vi "Multi Reader - Read Same Rates - State Machine.vi"(7 "Popup? (F)":bool, 8 "error in (no error)":errorcluster, 10 "Signals in":refnum<class "ISignal.lvclass">[](array[class])) -> (0 "error out":errorcluster)   [LabVIEW 2022 SP3, in "MultiReader.lvlib"]
uses:
  <instrlib>/openDAQ/Examples/MultiReader/MultiReader.lvlib
  <instrlib>/openDAQ/Public/TypeDef/DomainMetadata.ctl
  <instrlib>/openDAQ/Public/Classes/ISignal/ISignal.lvclass
  C:/Program Files (x86)/National Instruments/LabVIEW 2022/instr.lib/openDAQ/Public/Classes/IComponent/IComponent.lvclass
  C:/Program Files (x86)/National Instruments/LabVIEW 2022/instr.lib/openDAQ/Public/Classes/IBaseObject/IBaseObject.lvclass
  <instrlib>/openDAQ/Examples/MultiReader/TypeDef/State.ctl
  <instrlib>/openDAQ/Public/Classes/IInstance/IInstance.lvclass
  C:/Program Files (x86)/National Instruments/LabVIEW 2022/instr.lib/openDAQ/Public/Classes/IDevice/IDevice.lvclass
  <instrlib>/openDAQ/Public/Classes/IDevice/IDevice.lvclass
  <instrlib>/openDAQ/Public/Classes/IMultiReader/IMultiReader.lvclass
  C:/Program Files (x86)/National Instruments/LabVIEW 2022/instr.lib/openDAQ/Public/Classes/IReader/IReader.lvclass
  <instrlib>/openDAQ/Public/TypeDef/daqSampleType.ctl
  <instrlib>/openDAQ/Public/Classes/IMultiReaderStatus/IMultiReaderStatus.lvclass
  C:/Program Files (x86)/National Instruments/LabVIEW 2022/instr.lib/openDAQ/Public/Classes/IReaderStatus/IReaderStatus.lvclass
  <instrlib>/openDAQ/Public/Classes/IBaseObject/Polymorphic/queryInterface/queryDataDescriptorInterface.vi
  <instrlib>/openDAQ/Public/Classes/IMultiReaderBuilder/IMultiReaderBuilder.lvclass
  <instrlib>/openDAQ/Public/Classes/daqCoreTypes/IDict/IDict.lvclass
  <instrlib>/openDAQ/Public/Classes/IBaseObject/IBaseObject.lvclass
  <instrlib>/openDAQ/Public/Classes/IDataDescriptor/IDataDescriptor.lvclass
  <instrlib>/openDAQ/Public/Classes/IEventPacket/IEventPacket.lvclass
  <instrlib>/openDAQ/Public/Classes/daqUtils/daqUtils.lvlib
  <instrlib>/openDAQ/openDAQ.lvlib
  <instrlib>/openDAQ/Public/Classes/IComponent/IComponent.lvclass
  <instrlib>/openDAQ/Public/Classes/IReader/IReader.lvclass
  <instrlib>/openDAQ/Public/Classes/IReaderStatus/IReaderStatus.lvclass
panel:
  in  "Btn:StopMeasurement":bool
  in  "Online Buffer":i32=1000
  in  "Btn:StartMeasurement":bool
  out "Str:SampleRate":string
  in  "Btn:Stop":bool
  out "Iteration":i32
  out "DomainMetadata":T1
  out "Global ID's":string[](array[string])
  out "XY Graph":cluster{dbl[], "Read Buffers out":dbl[]}[](graph)
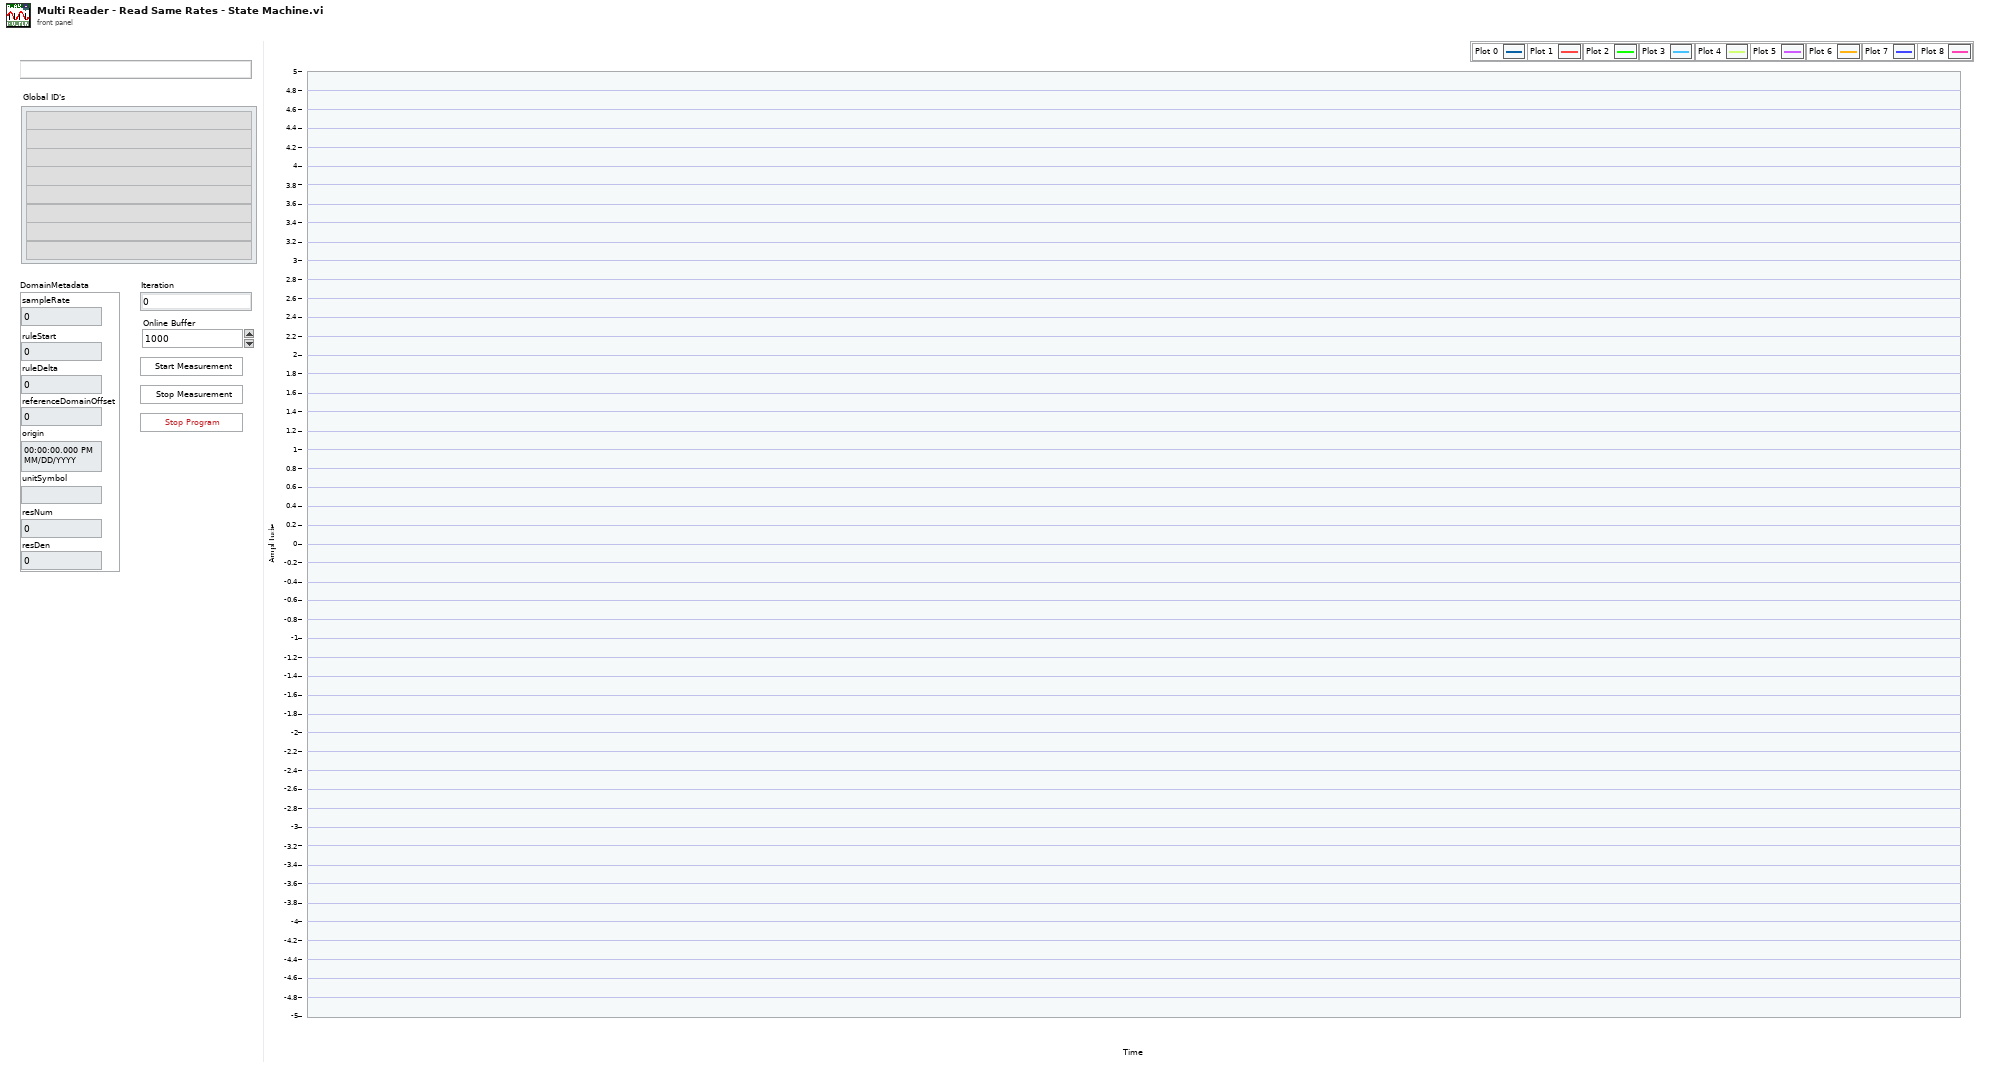
[diagram p1: front panel]
types:
  T1 = typedef "openDAQ.lvlib/DomainMetadata.ctl" = cluster{"sampleRate":i64, "ruleStart":i64, "ruleDelta":i64, "referenceDomainOffset":i64, "origin":timestamp, "unitSymbol":string, "resNum":i64, "resDen":i64}
  T2 = cluster{"Simulator":refnum<class "IInstance.lvclass">, "Instance":refnum<class "IInstance.lvclass">, "ConnectedDevice":refnum<class "IDevice.lvclass">, "Signals":refnum<class "ISignal.lvclass">[], "ChannelCount":i32, "MultiReader":refnum<class "IMultiReader.lvclass">}
  T3 = typedef "MultiReader.lvlib/State.ctl" = enum16{"INIT", "- SIMULATOR.setup", "IDLE", "- DAQ.start", "- DAQ.read", "- DAQ.end", "STOP", "ERROR"}
  T4 = enum16{"init", "read", "set sampleRate", "set ruleStart", "set ruleDelta", "set referenceDomainOffset", "set origin", "set unitSymbol", "set resNum", "set resDen", " calculate sampleRate"}
  T5 = enum8{"Enabled", "Disabled", "Disabled and Grayed Out"}
  T6 = typedef "openDAQ.lvlib/daqSampleType.ctl" = u16
  T7 = typedef "openDAQ.lvlib/ReadStatus.ctl" = u16
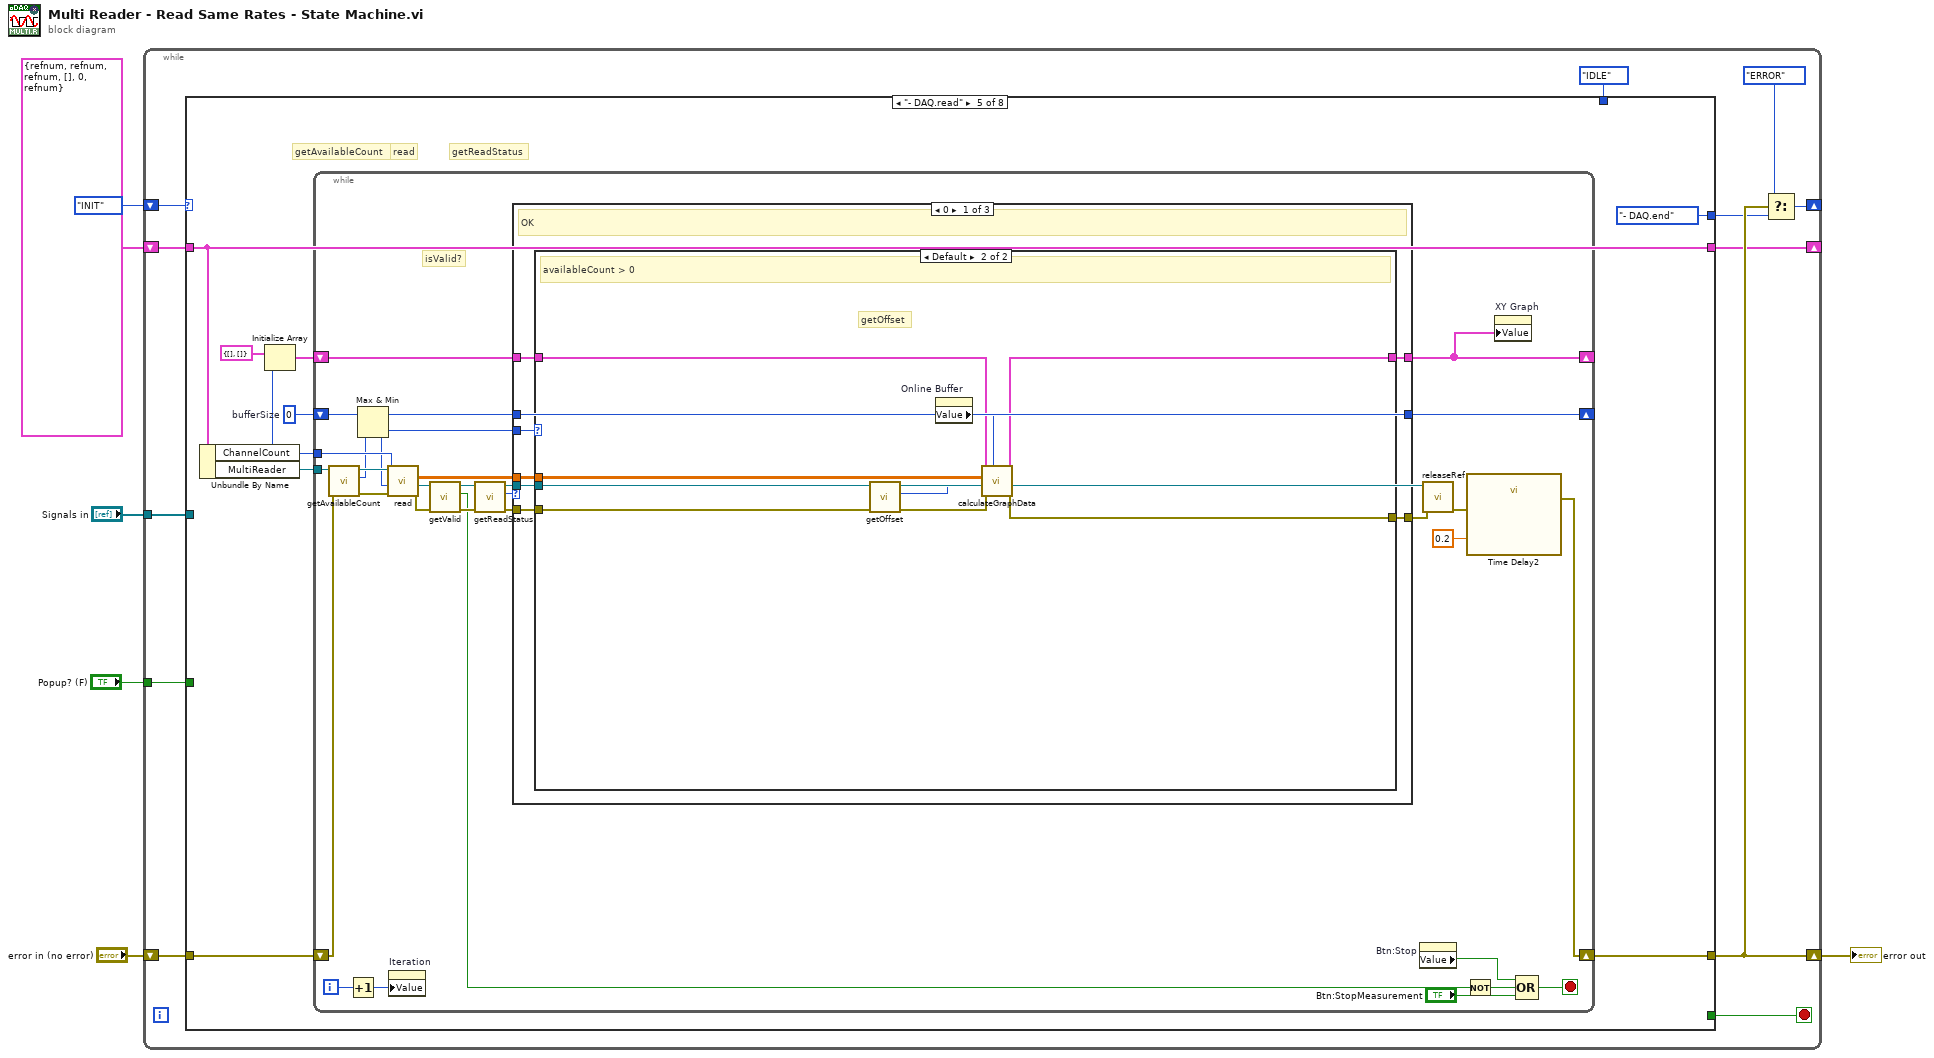
[diagram p0: block diagram]
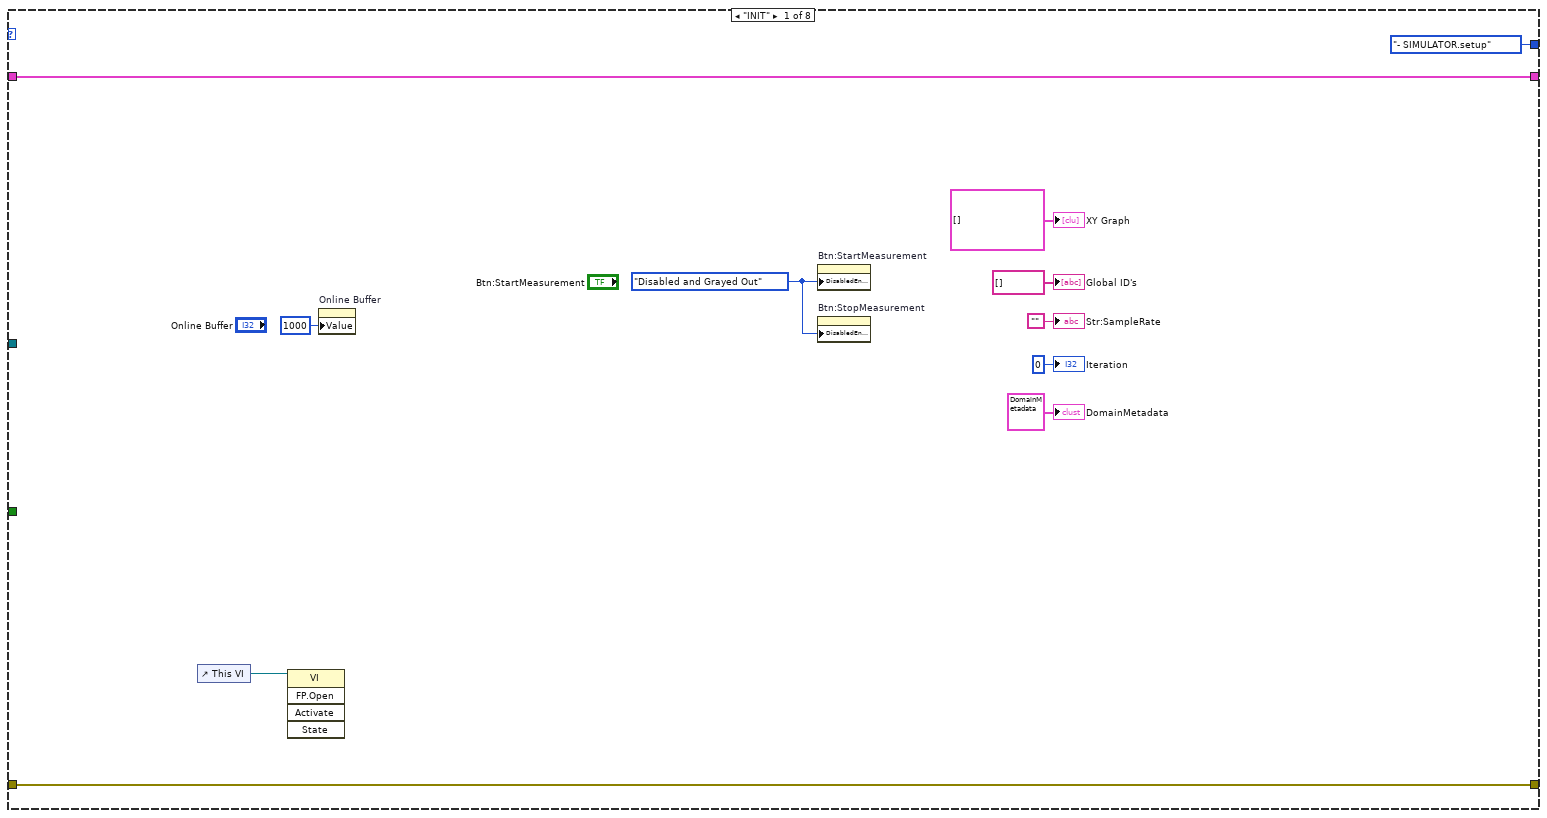
[diagram p2: hidden frame]
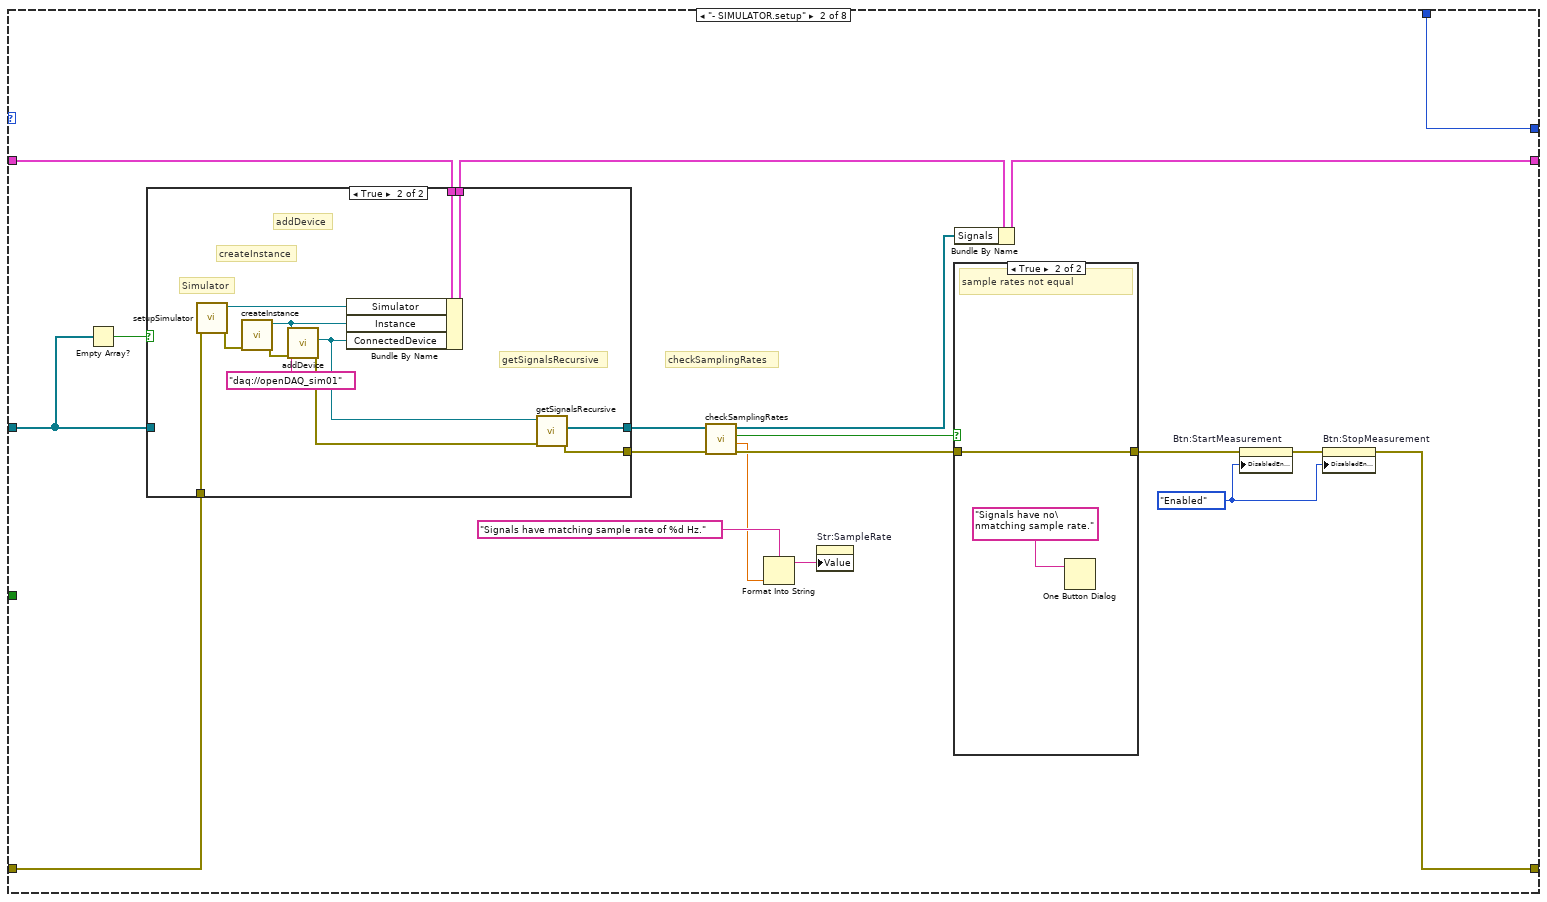
[diagram p3: hidden frame]
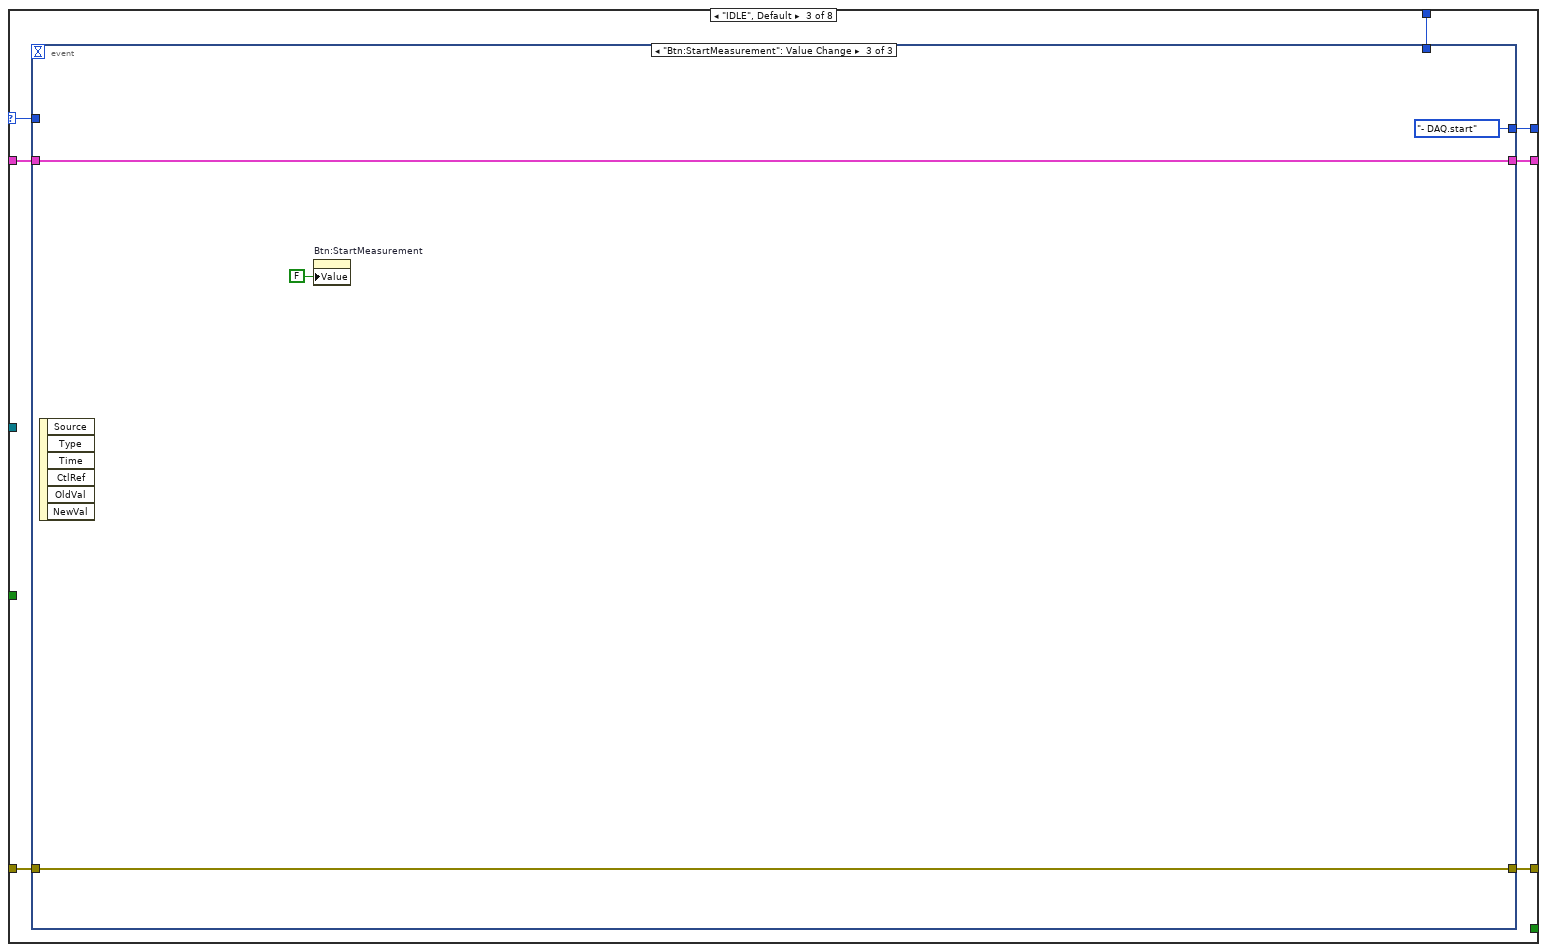
[diagram p6: hidden frame]
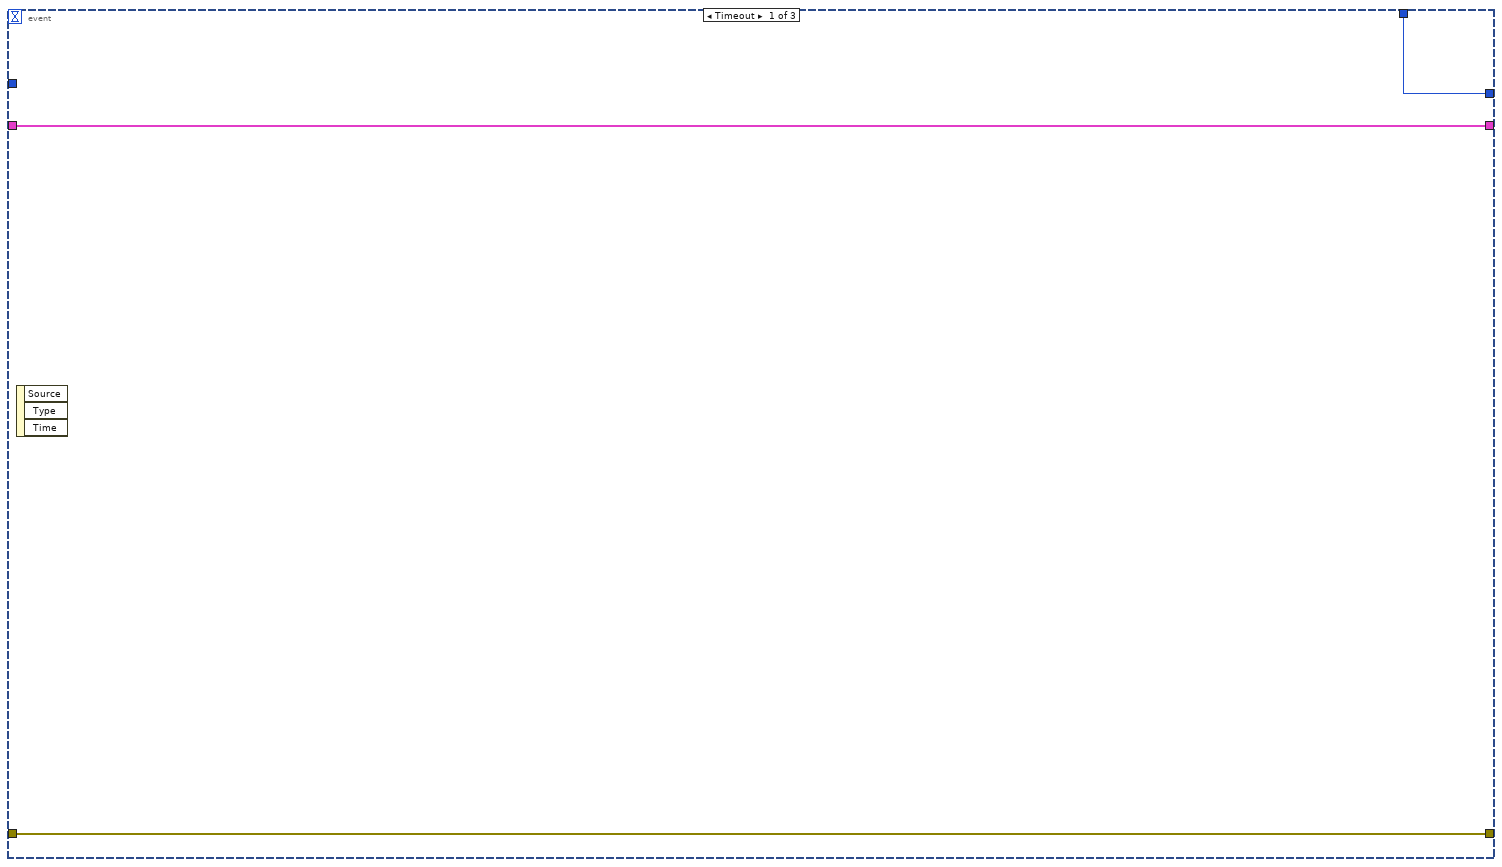
[diagram p7: hidden frame]
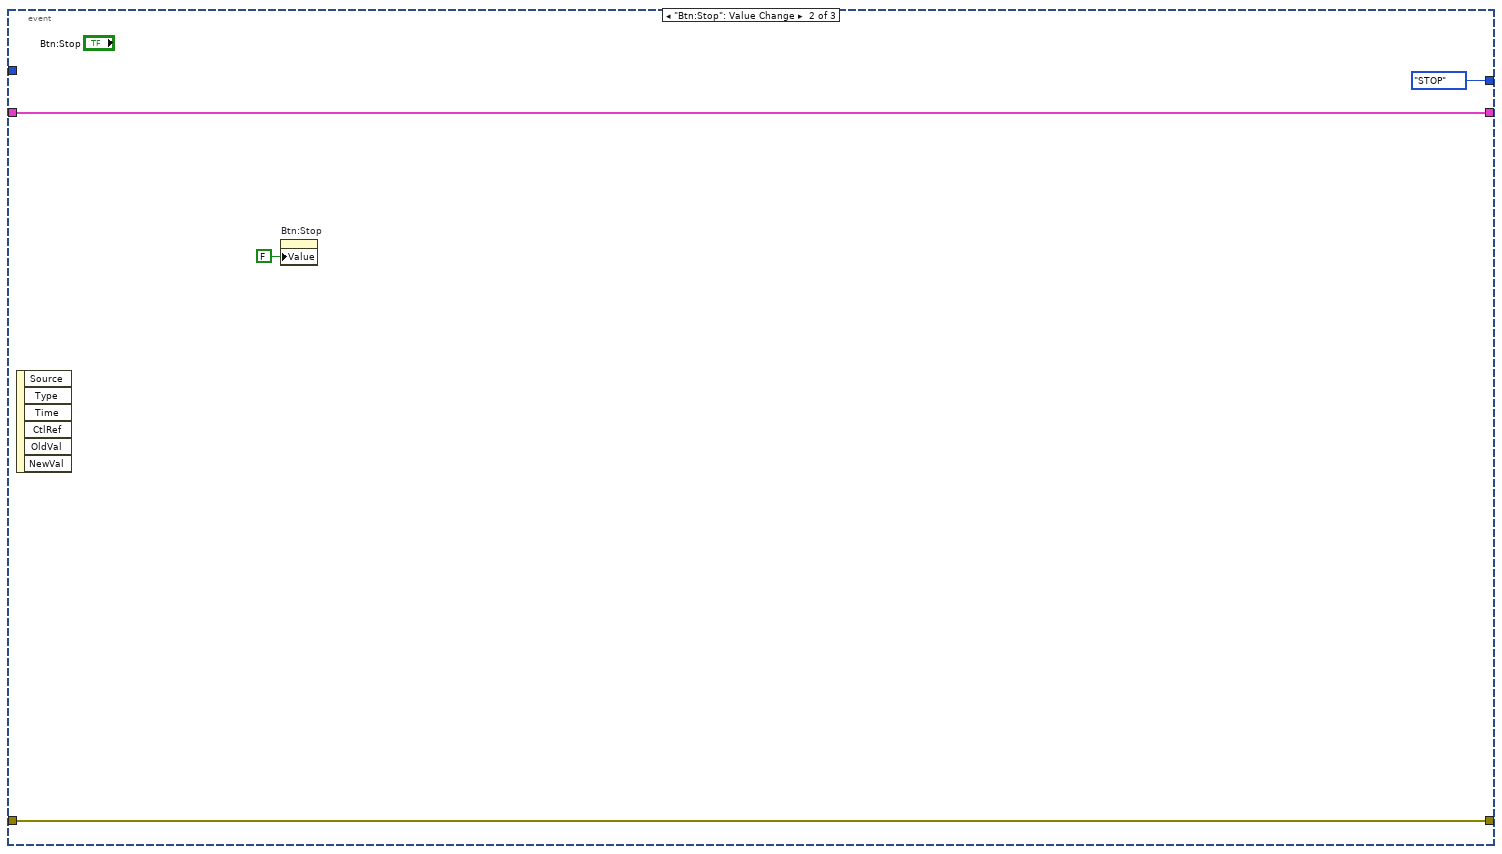
[diagram p8: hidden frame]
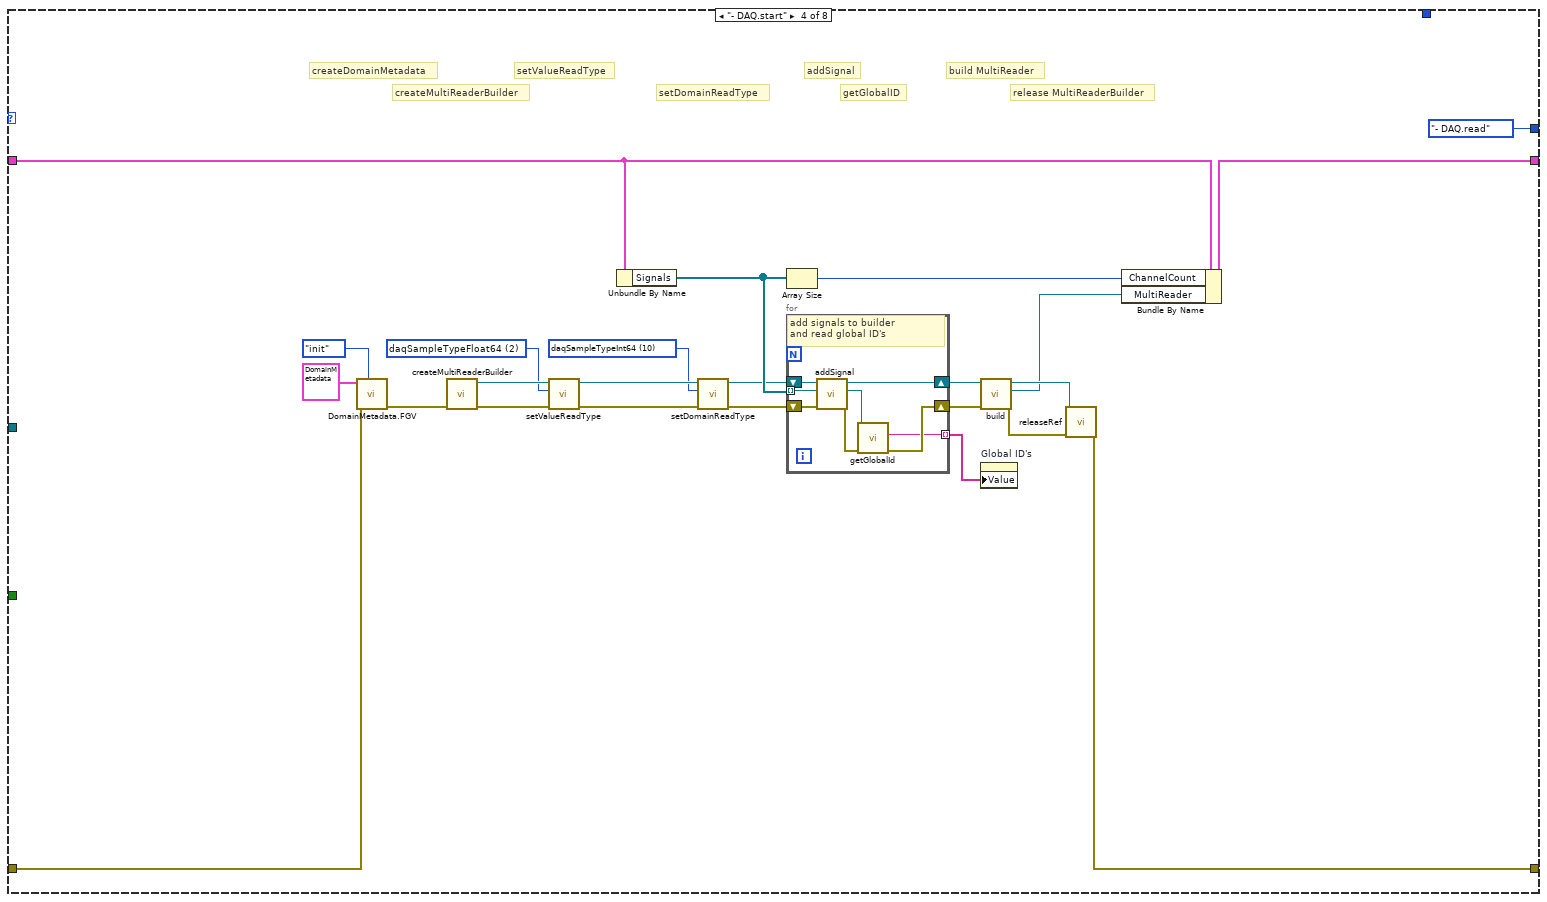
[diagram p9: hidden frame]
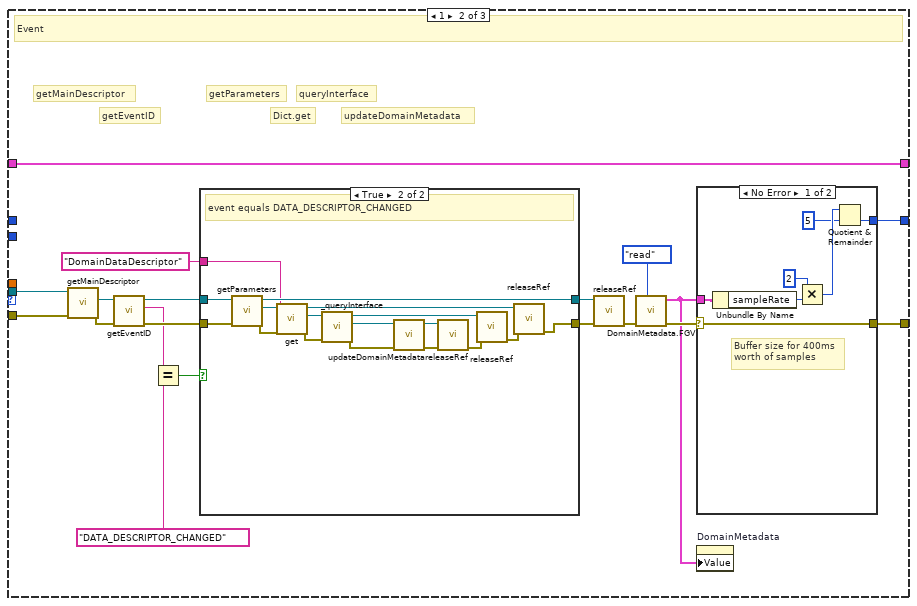
[diagram p11: hidden frame]
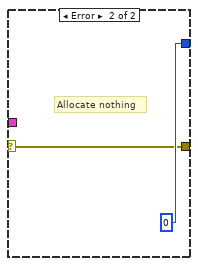
[diagram p12: hidden frame]
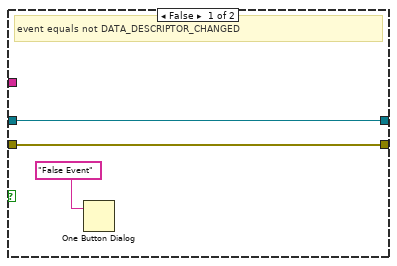
[diagram p13: hidden frame]
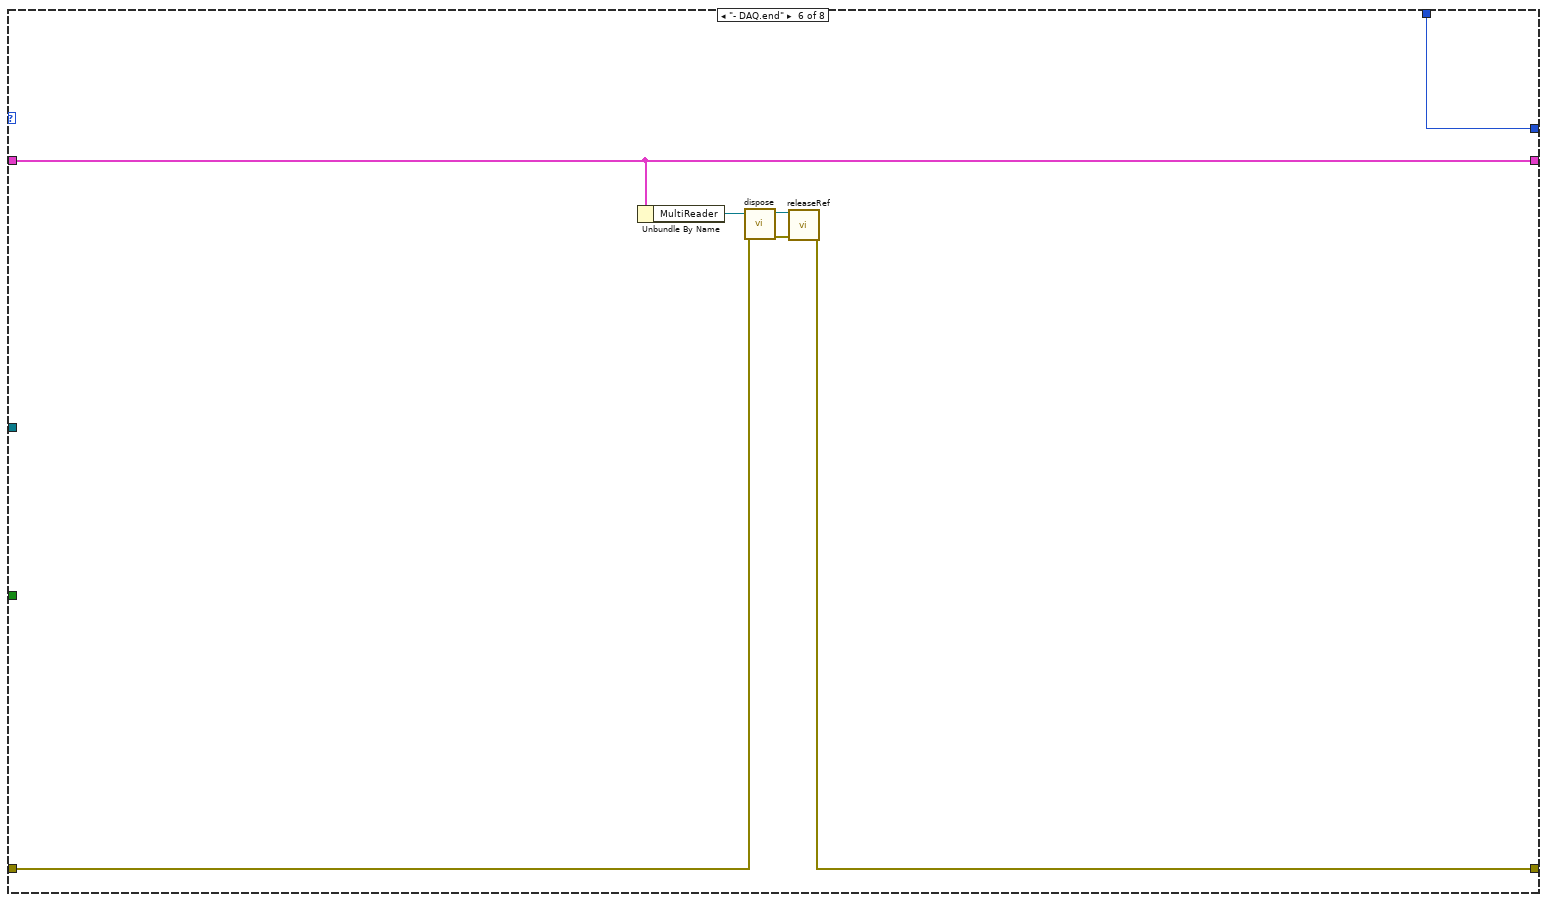
[diagram p15: hidden frame]
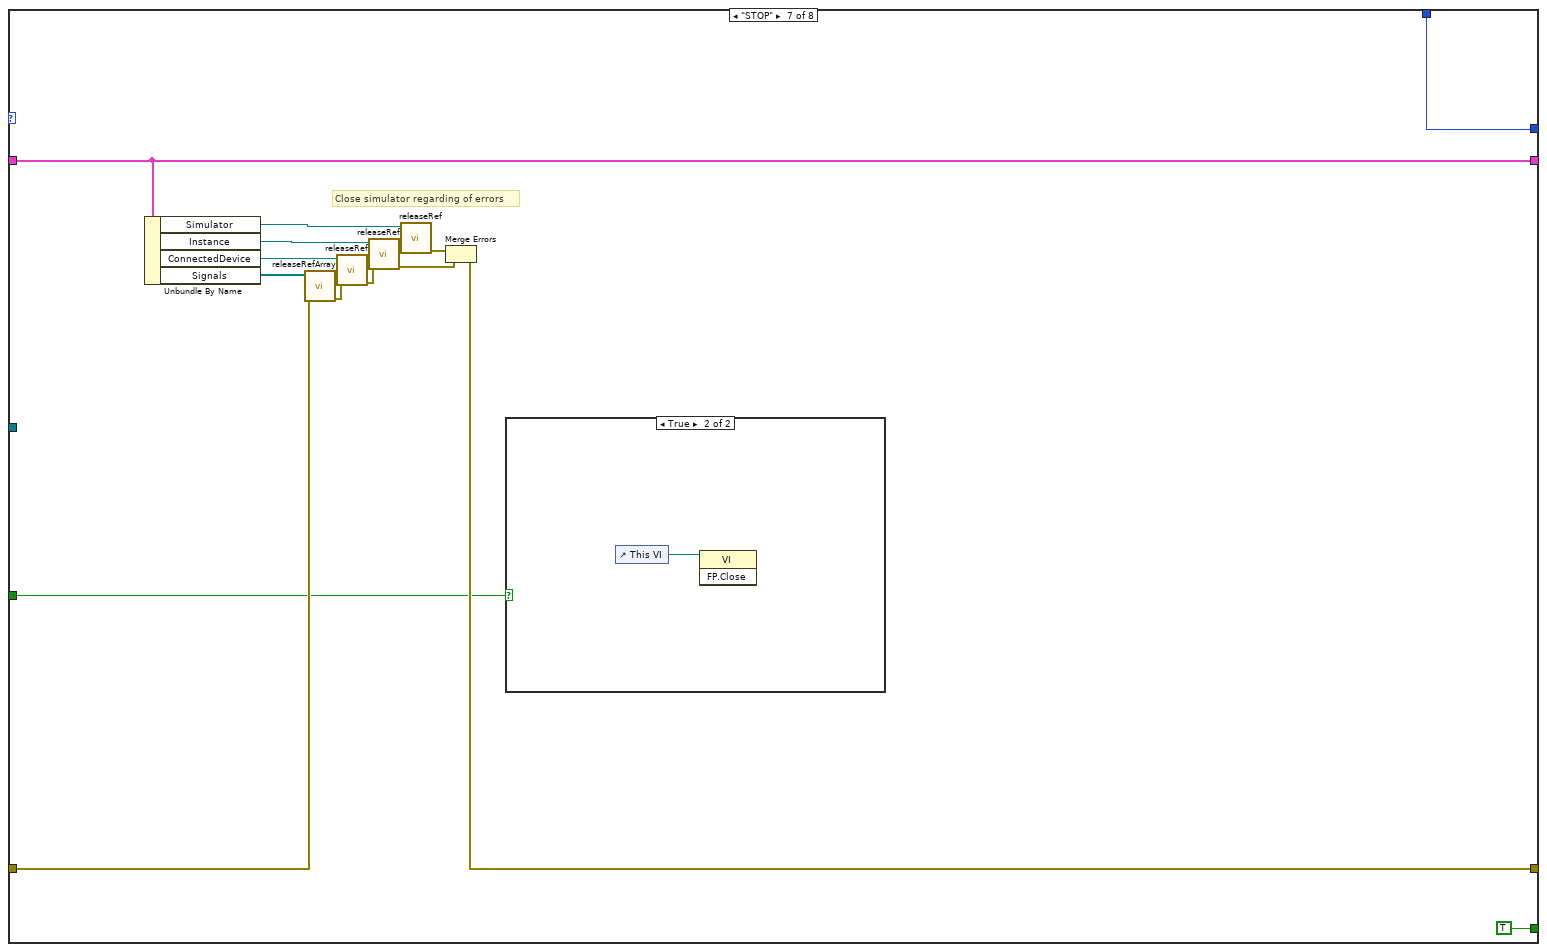
[diagram p16: hidden frame]
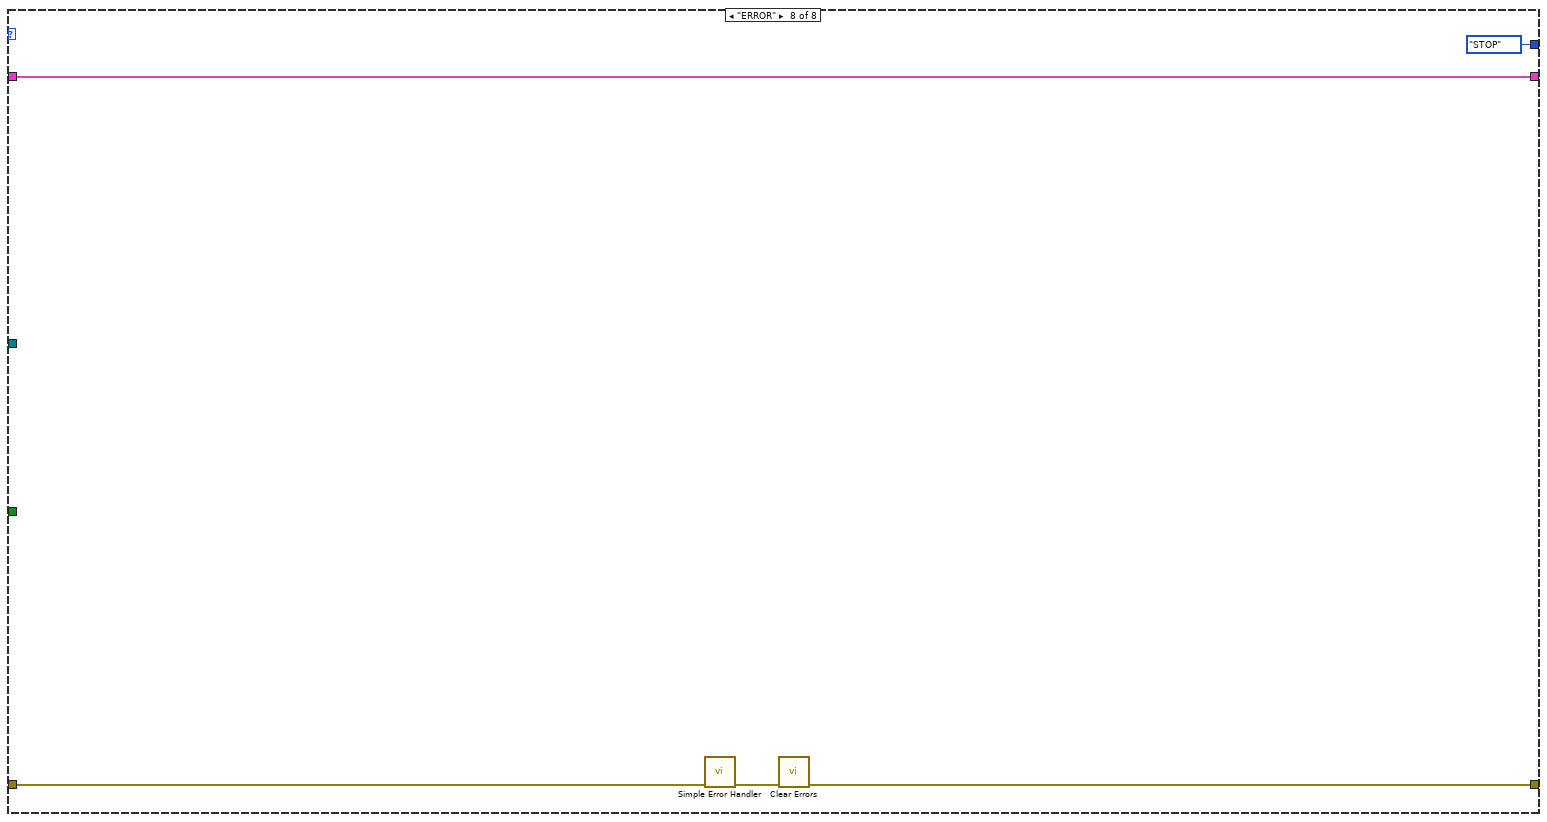
[diagram p18: hidden frame]
diagram:
  n1 = while {
    shift-right: [w11] -> _
    shift-left: State."INIT" -> [w17]
    shift-right: [w18] -> w2
    shift-left: "error in (no error)" -> [w14]
    shift-right: [w12] -> _
    shift-left: T2 {"Simulator"=refnum, "Instance"=refnum, "ConnectedDevice"=refnum, "Signals"=[], "ChannelCount"=0, "MultiReader"=refnum} -> [w13]
    tunnel: "Signals in" -> [w8]
    tunnel: "Popup? (F)" -> [w7]
    stop <- w16 stop-if-true
    n2 = case shown="\"- DAQ.read\"" w17 {
      selector: w17 -> [_ _ w73 _ _ _ _ _]
      tunnel: [State."- SIMULATOR.setup" w47 w71 State."- DAQ.read" State."- DAQ.end" w233 w235 State."STOP"] -> w10
      tunnel: [_ _ _ _ _ _ TRUE _] -> w16
      tunnel: State."IDLE" -> [_ w47 w72 _ _ w233 w235 _]
      tunnel: w14 -> [w22 w48 w70 w93 w123 w229 w237 w251]
      tunnel: [w22 w33 w69 w87 w122 w231 w240 w250] -> w18
      tunnel: w13 -> [w29 w46 w68 w97 w124 w232 w246 w253]
      tunnel: [w29 w41 w67 w85 w124 w232 w246 w253] -> w12
      tunnel: w8 -> [_ w30 _ _ _ _ _ _]
      tunnel: w7 -> [_ _ _ _ _ _ w234 _]
      frame "INIT" {
        w20 = T5."Disabled and Grayed Out" ("Disabled")
        n3 = control-ref of="This VI"() -> (w19:refnum<vi>)
        n4 = invoke class="VI" method="FP.Open"(reference=w19) -> ()  [unwired: 4 in, 5 out]
        n5 = property on="Online Buffer" class="DigNum (strict)"("Value"=1000 ("Online Buffer")) -> ()  [unwired: 2 in, 2 out]
        n6 = property on="Btn:StartMeasurement" class="Bool (strict)"("DisabledEnum"=w20) -> ()  [unwired: 2 in, 2 out]
        n7 = property on="Btn:StopMeasurement" class="Bool"("DisabledEnum"=w20) -> ()  [unwired: 2 in, 2 out]
        "Global ID's" <- string[] [] ("Global ID's")
        "Str:SampleRate" <- "" ("Str:SampleRate")
        "Iteration" <- 0 ("Iteration")
        "XY Graph" <- cluster{dbl[], "Read Buffers out":dbl[]}[] [] ("XY Graph")
        "DomainMetadata" <- T1 {"sampleRate"=0, "ruleStart"=0, "ruleDelta"=0, "referenceDomainOffset"=0, "origin"=timestamp(0 s since 1904-01-01), "unitSymbol"="", "resNum"=0, "resDen"=0} ("DomainMetadata")
      }
      frame "- SIMULATOR.setup" {
        w32 = T5."Enabled" ("Disabled")
        # "checkSamplingRates"
        n8 = Empty Array?(array=w30) -> (empty?=w31:bool)
        n9 = case shown="True" w31 {
          tunnel: w48 -> [w50 w63]
          tunnel: w46 -> [w51 w57]
          tunnel: [w49 w56] -> w45
          tunnel: [w51 w53] -> w42
          tunnel: [w50 w52] -> w36
          tunnel: w30 -> [w49 _]
          frame False {
          }
          frame True {
            # "Simulator"
            # "addDevice"
            # "createInstance"
            # "getSignalsRecursive"
            n10 = call <instrlib>:"setupSimulator.vi"("error in (no error)"=w63) -> ("error out"=w60:errorcluster, "IInstance out"=w59:refnum<class "IInstance.lvclass">)  [unwired: 9 in]
            n11 = call <instrlib>:"createInstance.vi"("error in (no error)"=w60) -> ("error out"=w62:errorcluster, "IInstance out"=w58:refnum<class "IInstance.lvclass">)  [unwired: 9 in]
            n12 = call <instrlib>:"addDevice.vi"("error in (no error)"=w62, "ConnectionString in"="daq://openDAQ_sim01" ("modulePath"), "IDevice in"=w58) -> ("error out"=w55:errorcluster, "ConnectedDevice out"=w54:refnum<class "IDevice.lvclass">)  [unwired: 6 in, 1 out]
            n13 = Bundle By Name(cluster=w57, "Simulator"=w59, "Instance"=w58, "ConnectedDevice"=w54) -> (w53:T2)
            n14 = call <instrlib>:"getSignalsRecursive.vi"("error in (no error)"=w55, "IDevice in"=w54) -> ("error out"=w52:errorcluster, "Available Sigals out"=w56:refnum<class "ISignal.lvclass">[])  [unwired: 7 in, 1 out]
          }
        }
        n15 = call <instrlib>:"checkSamplingRates.vi"("error in (no error)"=w36, "Available Sigals in"=w45) -> ("error out"=w44:errorcluster, "SampleRate"=w39:dbl, "Boolean"=w43:bool, "Array"=w37:refnum<class "ISignal.lvclass">[])  [unwired: 6 in]
        n16 = Format Into String(format string="Signals have matching sample rate of %d Hz.", w39) -> (resulting string=w38:string)  [unwired: 2 in, 1 out]
        n17 = property on="Str:SampleRate" class="Str"("Value"=w38) -> ()  [unwired: 2 in, 2 out]
        n18 = case shown="True" w43 {
          tunnel: w44 -> [w64 w66]
          tunnel: [w64 w66] -> w35
          frame False {
            # "all sample rates are equal"
          }
          frame True {
            # "sample rates not equal"
            n19 = One Button Dialog(message="Signals have no\nmatching sample rate.") -> ()  [unwired: 1 in, 1 out]
          }
        }
        n20 = Bundle By Name(cluster=w42, "Signals"=w37) -> (w41:T2)
        n21 = property on="Btn:StartMeasurement" class="Bool (strict)"(error in=w35, "DisabledEnum"=w32) -> (error out=w34:errorcluster)  [unwired: 1 in, 1 out]
        n22 = property on="Btn:StopMeasurement" class="Bool"(error in=w34, "DisabledEnum"=w32) -> (error out=w33:errorcluster)  [unwired: 1 in, 1 out]
      }
      frame "IDLE", Default {
        n23 = event shown="[2] \"Btn:StartMeasurement\": Value Change" {
          selector: _ -> [_ _ _]
          dyn-events: _ -> [_ _ _]
          timeout: _ -> [_ _ _]
          tunnel: w73 -> [_ _ _]
          tunnel: [w76 State."STOP" State."- DAQ.start"] -> w71
          tunnel: w72 -> [w76 _ _]
          tunnel: w70 -> [w75 w80 w82]
          tunnel: [w75 w80 w82] -> w69
          tunnel: w68 -> [w74 w79 w83]
          tunnel: [w74 w79 w83] -> w67
          event Timeout {
            n24 = event-data() -> ()  [unwired: 1 in, 3 out]
          }
          event "Btn:Stop": Value Change {
            n25 = event-data() -> ()  [unwired: 1 in, 6 out]
            n26 = property on="Btn:Stop" class="Bool (strict)"("Value"=FALSE ("Btn:Stop")) -> ()  [unwired: 2 in, 2 out]
          }
          event "Btn:StartMeasurement": Value Change {
            n27 = event-data() -> ()  [unwired: 1 in, 6 out]
            n28 = property on="Btn:StartMeasurement" class="Bool (strict)"("Value"=FALSE ("Btn:StartMeasurement")) -> ()  [unwired: 2 in, 2 out]
          }
        }
      }
      frame "- DAQ.start" {
        w103 = T6 10 items=["daqSampleTypeInvalid", "daqSampleTypeFloat32", "daqSampleTypeFloat64", "daqSampleTypeUInt8", "daqSampleTypeInt8", "daqSampleTypeUInt16", "daqSampleTypeInt16", "daqSampleTypeUInt32", "daqSampleTypeInt32", "daqSampleTypeUInt64", "daqSampleTypeInt64", "daqSampleTypeRangeInt64", "daqSampleTypeComplexFloat32", "daqSampleTypeComplexFloat64", "daqSampleTypeBinary", "daqSampleTypeString", "daqSampleTypeStruct", "daqSampleTypeNull", "daqSampleType_count"] ("daqSampleType")
        w106 = T6 2 items=["daqSampleTypeInvalid", "daqSampleTypeFloat32", "daqSampleTypeFloat64", "daqSampleTypeUInt8", "daqSampleTypeInt8", "daqSampleTypeUInt16", "daqSampleTypeInt16", "daqSampleTypeUInt32", "daqSampleTypeInt32", "daqSampleTypeUInt64", "daqSampleTypeInt64", "daqSampleTypeRangeInt64", "daqSampleTypeComplexFloat32", "daqSampleTypeComplexFloat64", "daqSampleTypeBinary", "daqSampleTypeString", "daqSampleTypeStruct", "daqSampleTypeNull", "daqSampleType_count"] ("daqSampleType")
        # "release MultiReaderBuilder"
        # "build MultiReader"
        # "createDomainMetadata"
        # "getGlobalID"
        # "addSignal"
        # "setDomainReadType"
        # "setValueReadType"
        # "createMultiReaderBuilder"
        n29 = call <instrlib>:"DomainMetadata.FGV.vi"("Case Select"=T4."init", "error in"=w93, "DomainMetadata in"=T1 {"sampleRate"=1, "ruleStart"=0, "ruleDelta"=1, "referenceDomainOffset"=0, "origin"=timestamp(0 s since 1904-01-01), "unitSymbol"="", "resNum"=0, "resDen"=0}) -> ("error out"=w102:errorcluster)  [unwired: 7 in, 1 out]
        n30 = call <instrlib>:"createMultiReaderBuilder.vi"("error in (no error)"=w102) -> ("error out"=w108:errorcluster, "IMultiReaderBuilder out"=w107:refnum<class "IMultiReaderBuilder.lvclass">)  [unwired: 9 in]
        n31 = call <instrlib>:"setValueReadType.vi"("error in (no error)"=w108, "SampleType in"=w106, "IMultiReaderBuilder in"=w107) -> ("error out"=w104:errorcluster, "IMultiReaderBuilder out"=w105:refnum<class "IMultiReaderBuilder.lvclass">)  [unwired: 7 in]
        n32 = Unbundle By Name(w97) -> ("Signals"=w95:refnum<class "ISignal.lvclass">[])
        n33 = call <instrlib>:"setDomainReadType.vi"("error in (no error)"=w104, "SampleType in"=w103, "IMultiReaderBuilder in"=w105) -> ("error out"=w98:errorcluster, "IMultiReaderBuilder out"=w94:refnum<class "IMultiReaderBuilder.lvclass">)  [unwired: 7 in]
        n34 = Array Size(array=w95) -> (size(s)=w96:i32)
        n35 = for {
          tunnel: w95 -> [w113] mode=indexing
          shift-right: [w112] -> w90
          shift-left: w94 -> [w115]
          shift-right: [w116] -> w92
          shift-left: w98 -> [w114]
          tunnel: [w109] -> w86 mode=indexing
          # "add signals to builder\nand read global ID's"
          n36 = call <instrlib>:"addSignal.vi"("error in (no error)"=w114, "ISignal in"=w113, "IMultiReaderBuilder in"=w115) -> ("error out"=w111:errorcluster, "ISignal out"=w110:refnum<class "ISignal.lvclass">, "IMultiReaderBuilder out"=w112:refnum<class "IMultiReaderBuilder.lvclass">)  [unwired: 5 in, 1 out]
          n37 = call <instrlib>:"getGlobalId.vi"("error in (no error)"=w111, "IComponent in"=w110) -> ("error out"=w116:errorcluster, "GlobalId out"=w109:string)  [unwired: 7 in, 1 out]
        }
        n38 = call <instrlib>:"build.vi"("error in (no error)"=w92, "IMultiReaderBuilder in"=w90) -> ("error out"=w91:errorcluster, "IMultiReader out"=w88:refnum<class "IMultiReader.lvclass">, "IMultiReaderBuilder out"=w89:refnum<class "IMultiReaderBuilder.lvclass">)  [unwired: 6 in, 1 out]
        n39 = property on="Global ID's" class="Arr (strict)"("Value"=w86) -> ()  [unwired: 2 in, 2 out]
        n40 = call-dynamic "releaseRef.vi"("error in (no error)"=w91, "IBaseObject in"=w89) -> ("error out"=w87:errorcluster)  [unwired: 9 in]
        n41 = Bundle By Name(cluster=w97, "ChannelCount"=w96, "MultiReader"=w88) -> (w85:T2)
      }
      frame "- DAQ.read" {
        w117 = i64 0  # bufferSize
        # "getReadStatus"
        # "read"
        # "getAvailableCount"
        n42 = Unbundle By Name(w124) -> ("ChannelCount"=w118:i32, "MultiReader"=w121:refnum<class "IMultiReader.lvclass">)
        n43 = Initialize Array(cluster{dbl[], dbl[]} {[], []}, w118) -> (w119:cluster{dbl[], dbl[]}[])
        n44 = while {
          shift-right: [w141] -> w122
          shift-left: w123 -> [w145]
          tunnel: w121 -> [w155]
          shift-right: [w135] -> _
          shift-left: w119 -> [w136]
          tunnel: w118 -> [w153]
          shift-right: [w139] -> _
          shift-left: w117 -> [w151]
          i -> [w150]
          stop <- w127 stop-if-true
          # "isValid?"
          n45 = call <instrlib>:"getAvailableCount.vi"("error in (no error)"=w145, "IReader in"=w155) -> ("error out"=w156:errorcluster, "Available Count"=w152:i32, "IReader out"=w154:refnum<class "IMultiReader.lvclass">)  [unwired: 7 in]
          n46 = Increment(x=w150) -> (x+1=w149:i32)
          n47 = Max & Min(x=w151, y=w152) -> (max(x,y)=w138:i64, min(x,y)=w137:i64)
          n48 = call <instrlib>:"read.vi"("error in (no error)"=w156, "bufferSize"=w137, "signalCount"=w153, "IMultiReader in"=w154) -> ("error out"=w134:errorcluster, "Multi Reader Status out"=w132:refnum<class "IMultiReaderStatus.lvclass">, "Read Buffers out"=w146:dbl[][])  [unwired: 4 in, 1 out]
          n49 = property on="Iteration" class="DigNum (strict)"("Value"=w149) -> ()  [unwired: 2 in, 2 out]
          n50 = call <instrlib>:"getValid.vi"("error in (no error)"=w134, "ReaderStatus in"=w132) -> ("error out"=w133:errorcluster, "isValid?"=w130:bool, "ReaderStatus out"=w131:refnum<class "IMultiReaderStatus.lvclass">)  [unwired: 7 in]
          n51 = call <instrlib>:"getReadStatus.vi"("error in (no error)"=w133, "IReaderStatus in"=w131) -> ("error out"=w147:errorcluster, "ReadStatus"=w148:T7, "IReaderStatus out"=w144:refnum<class "IMultiReaderStatus.lvclass">)  [unwired: 7 in]
          n52 = case shown="0" w148 {
            tunnel: w147 -> [w161 w192 w226]
            tunnel: w144 -> [w162 w193 _]
            tunnel: w146 -> [w160 _ _]
            tunnel: [w157 w179 w226] -> w143
            tunnel: [w164 w178 w225] -> w139
            tunnel: w138 -> [w164 _ w225]
            tunnel: w137 -> [w163 _ _]
            tunnel: w136 -> [w159 w177 w224]
            tunnel: [w158 w177 w224] -> w135
            frame 0 {
              # "OK"
              n53 = case shown="Default" w163 {
                tunnel: w162 -> [_ w175]
                tunnel: w161 -> [w165 w174]
                tunnel: w160 -> [_ w173]
                tunnel: w159 -> [w166 w172]
                tunnel: [w166 w169] -> w158
                tunnel: [w165 w168] -> w157
                frame 0 {
                  # "availableCount = 0"
                }
                frame Default {
                  # "getOffset"
                  # "availableCount > 0"
                  n54 = call <instrlib>:"getOffset.vi"("error in (no error)"=w174, "IReaderStatus in"=w175) -> ("error out"=w171:errorcluster, "Offset out"=w170:i64)  [unwired: 7 in, 1 out]
                  n55 = property on="Online Buffer" class="DigNum (strict)"() -> ("Value"=w167:i32)  [unwired: 2 in, 2 out]
                  n56 = call <instrlib>:"calculateGraphData.vi"("Online Buffer (1000)"=w167, "error in"=w171, "Offset in"=w170, "DataBuffers in"=w173, "GraphData in"=w172) -> ("error out"=w168:errorcluster, "GraphData out"=w169:cluster{dbl[], dbl[]}[])  [unwired: 5 in]
                }
              }
            }
            frame 1 {
              # "updateDomainMetadata"
              # "Dict.get"
              # "queryInterface"
              # "getParameters"
              # "getEventID"
              # "getMainDescriptor"
              # "Event"
              n57 = call <instrlib>:"getMainDescriptor.vi"("error in (no error)"=w192, "IMultiReaderStatus in"=w193) -> ("error out"=w190:errorcluster, "EventPacket out"=w191:refnum<class "IEventPacket.lvclass">)  [unwired: 7 in, 1 out]
              n58 = call <instrlib>:"getEventID.vi"("error in (no error)"=w190, "IEventPacket in"=w191) -> ("error out"=w194:errorcluster, "EventID out"=w189:string, "IEventPacket out"=w187:refnum<class "IEventPacket.lvclass">)  [unwired: 7 in]
              n59 = Equal?(x=w189, y="DATA_DESCRIPTOR_CHANGED" ("x")) -> (x = y?=w188:bool)
              n60 = case shown="True" w188 {
                tunnel: w194 -> [w205 w222]
                tunnel: [w205 w207] -> w186
                tunnel: [w204 w221] -> w185
                tunnel: w187 -> [w204 w223]
                tunnel: "DomainDataDescriptor" -> [_ w216]
                frame False {
                  # "event equals not DATA_DESCRIPTOR_CHANGED"
                  n61 = One Button Dialog(message="False Event" ("x")) -> ()  [unwired: 1 in, 1 out]
                }
                frame True {
                  # "event equals DATA_DESCRIPTOR_CHANGED"
                  n62 = call <instrlib>:"getParameters.vi"("error in (no error)"=w222, "IEventPacket in"=w223) -> ("error out"=w217:errorcluster, "Parameters out"=w220:refnum<class "IDict.lvclass">, "IEventPacket out"=w221:refnum<class "IEventPacket.lvclass">)  [unwired: 7 in]
                  n63 = call <instrlib>:"get.vi"("error in (no error)"=w217, "Key in"=w216, "IDict in"=w220) -> ("error out"=w218:errorcluster, "Value out"=w219:refnum<class "IBaseObject.lvclass">, "IDict out"=w211:refnum<class "IDict.lvclass">)  [unwired: 6 in]
                  n64 = call-poly <instrlib>:"_queryInterface.vi"("error in (no error)"=w218, "IBaseObject in"=w219) -> ("error out"=w215:errorcluster, "DataDescriptor out"=w214:refnum<class "IDataDescriptor.lvclass">, "IBaseObject out"=w210:refnum<class "IBaseObject.lvclass">)  [unwired: 7 in]
                  n65 = call <instrlib>:"updateDomainMetadata.vi"("error in"=w215, "IDataDescriptor in"=w214) -> ("error out"=w212:errorcluster, "IDataDescriptor out"=w213:refnum<class "IDataDescriptor.lvclass">)  [unwired: 8 in]
                  n66 = call-dynamic "releaseRef.vi"("error in (no error)"=w212, "IBaseObject in"=w213) -> ("error out"=w209:errorcluster)  [unwired: 9 in]
                  n67 = call-dynamic "releaseRef.vi"("error in (no error)"=w209, "IBaseObject in"=w210) -> ("error out"=w208:errorcluster)  [unwired: 9 in]
                  n68 = call-dynamic "releaseRef.vi"("error in (no error)"=w208, "IBaseObject in"=w211) -> ("error out"=w207:errorcluster)  [unwired: 9 in]
                }
              }
              n69 = call-dynamic "releaseRef.vi"("error in (no error)"=w186, "IBaseObject in"=w185) -> ("error out"=w180:errorcluster)  [unwired: 9 in]
              n70 = call <instrlib>:"DomainMetadata.FGV.vi"("Case Select"=T4."read", "error in"=w180) -> ("error out"=w182:errorcluster, "DomainMetadata out"=w176:T1)  [unwired: 8 in]
              n71 = case shown="No Error" w182 {
                selector: w182 -> [w195 w202]
                tunnel: w176 -> [w201 _]
                tunnel: [w196 0] -> w178
                tunnel: [w195 w202] -> w179
                frame No Error {
                  # "Buffer size for 400ms\nworth of samples"
                  n72 = Unbundle By Name(w201) -> ("sampleRate"=w200:i64)
                  n73 = Multiply(x=2 ("y"), y=w200) -> (x*y=w198:i64)
                  n74 = Quotient & Remainder(x=w198, y=5) -> (floor(x/y)=w196:i64)  [unwired: 1 out]
                }
                frame Error {
                  # "Allocate nothing"
                }
              }
              n75 = property on="DomainMetadata" class="Clust (strict)"("Value"=w176) -> ()  [unwired: 2 in, 2 out]
            }
            frame Default {
              # "Failed, Unknown"
            }
          }
          n76 = property on="Btn:Stop" class="Bool (strict)"() -> ("Value"=w126:bool)  [unwired: 2 in, 2 out]
          n77 = call-dynamic "releaseRef.vi"("error in (no error)"=w143, "IBaseObject in"=w144) -> ("error out"=w142:errorcluster)  [unwired: 9 in]
          n78 = Not(x=w130) -> (.not. x?=w129:bool)
          n79 = call "Time Delay2"("error in (no error)"=w142, "Delay Time (s)"=0.2) -> ("error out"=w141:errorcluster)  [unwired: 9 in]
          n80 = property on="XY Graph" class="XYGraph (strict)"("Value"=w135) -> ()  [unwired: 2 in, 2 out]
          n81 = Compound Arithmetic op=OR(w126, w129, "Btn:StopMeasurement") -> (w127:bool)
        }
      }
      frame "- DAQ.end" {
        n82 = Unbundle By Name(w232) -> ("MultiReader"=w228:refnum<class "IMultiReader.lvclass">)
        n83 = call-dynamic "dispose.vi"("error in (no error)"=w229, "IBaseObject in"=w228) -> ("error out"=w230:errorcluster, "IBaseObject out"=w227:refnum<class "IBaseObject.lvclass">)  [unwired: 8 in]
        n84 = call-dynamic "releaseRef.vi"("error in (no error)"=w230, "IBaseObject in"=w227) -> ("error out"=w231:errorcluster)  [unwired: 9 in]
      }
      frame "STOP" {
        # "Close simulator regarding of errors"
        n85 = Unbundle By Name(w246) -> ("Simulator"=w243:refnum<class "IInstance.lvclass">, "Instance"=w244:refnum<class "IInstance.lvclass">, "ConnectedDevice"=w245:refnum<class "IDevice.lvclass">, "Signals"=w238:refnum<class "ISignal.lvclass">[])
        n86 = call <instrlib>:"releaseRefArray.vi"("error in (no error)"=w237, "IBaseObject in"=w238) -> ("error out"=w236:errorcluster)  [unwired: 9 in]
        n87 = call-dynamic "releaseRef.vi"("error in (no error)"=w236, "IBaseObject in"=w245) -> ("error out"=w242:errorcluster)  [unwired: 9 in]
        n88 = call-dynamic "releaseRef.vi"("error in (no error)"=w242, "IBaseObject in"=w244) -> ("error out"=w239:errorcluster)  [unwired: 9 in]
        n89 = call-dynamic "releaseRef.vi"("IBaseObject in"=w243) -> ("error out"=w241:errorcluster)  [unwired: 10 in]
        n90 = Merge Errors(w241, w239) -> (w240:errorcluster)
        n91 = case shown="True" w234 {
          frame False {
          }
          frame True {
            n92 = control-ref of="This VI"() -> (w248:refnum<vi>)
            n93 = invoke class="VI" method="FP.Close"(reference=w248) -> ()  [unwired: 2 in, 3 out]
          }
        }
      }
      frame "ERROR" {
        n94 = call <vilib>:"Simple Error Handler.vi"("error in (no error)"=w251) -> ("error out"=w252:errorcluster)  [unwired: 4 in, 4 out]
        n95 = call <vilib>:"Clear Errors.vi"("error in (no error)"=w252) -> ("error out"=w250:errorcluster)  [unwired: 5 in, 1 out]
      }
    }
    n96 = Select(t=State."ERROR", s=w18, f=w10) -> (s? t:f=w11:T3)
  }
  "error out" <- w2
